vi "Proceed.vi"(7 "component is ready (Y)":bool=TRUE, 8 "error in (no error)":errorcluster, 10 "ProceedMessage":refnum<class "ProceedMessage.lvclass">, 11 "ImageStack in":refnum<class "Invivo_ImageStack.lvclass">) -> (0 "error out":errorcluster, 2 "all observers are ready?":bool, 3 "ImageStack out":refnum<class "Invivo_ImageStack.lvclass">)   [LabVIEW 2012, in "Invivo_ImageStack.lvclass"]
uses:
  Invivo_ImageStack.lvclass
  <vilib>/Distrio/Murmex/ProceedMessage/ProceedMessage.lvclass
  Invivo_ImageStack.lvclass/Invivo_ImageStack.ctl
  <vilib>/Distrio/Murmex/Murmex/Murmex.lvclass
  <vilib>/Distrio/Murmex/Message/Message.lvclass
panel:
  # "This method is called when the PROCEED\ntrigger is sent. \n\nOverride this method when your component needs to\nrespond to this trigger. \n\nCall parent for proper implementation"
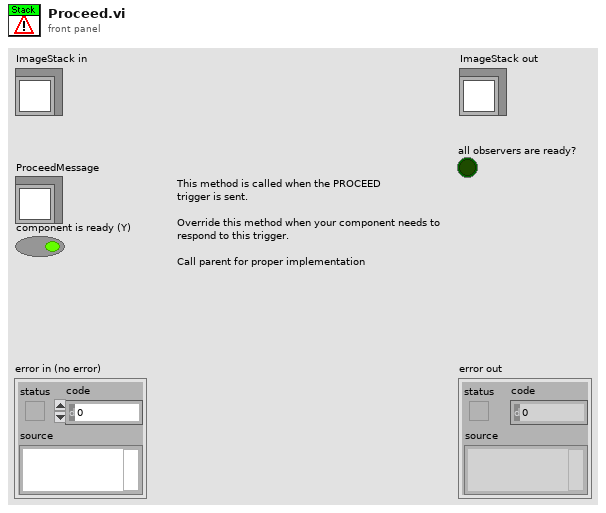
[diagram p1: front panel]
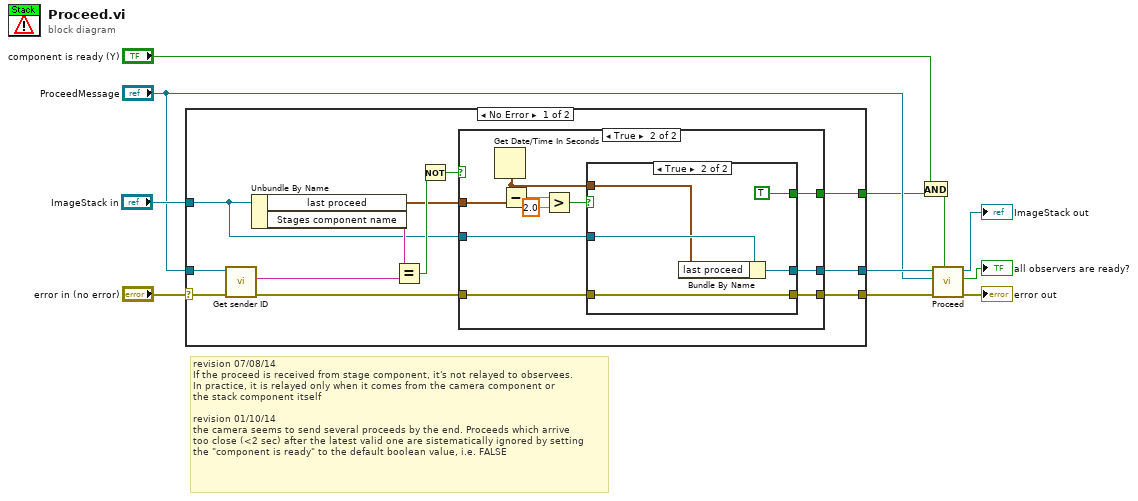
[diagram p0: block diagram]
diagram:
  # "revision 07/08/14\nIf the proceed is received from stage component, it's not relayed to observees.\nIn practice, it is relayed only when it comes from the camera component or \nthe stack component itself\n\nrevision 01/10/14\nthe camera seems to send several proceeds by the end. Proceeds which arrive\ntoo close (<2 sec) after the latest valid one are sistematically ignored by setting\nthe \"component is ready\" to the default boolean value, i.e. FALSE"
  n1 = case shown="No Error" "error in (no error)" {
    selector: "error in (no error)" -> [w22 w43]
    tunnel: "ImageStack in" -> [w15 w44]
    tunnel: [w12 w43] -> w6
    tunnel: [w13 w44] -> w5
    tunnel: "ProceedMessage" -> [w23 _]
    tunnel: [w14 _] -> w3
    frame No Error {
      n2 = call <vilib>:"Get sender ID.vi"("error in (no error)"=w22, "Message in"=w23) -> ("error out"=w17:errorcluster, "sender"=w21:string)  [unwired: 7 in, 1 out]
      n3 = Unbundle By Name(w15) -> ("last proceed"=w16:timestamp, "Stages component name"=w20:string)
      n4 = Equal?(x=w20, y=w21) -> (x = y?=w19:bool)
      n5 = Not(x=w19) -> (.not. x?=w18:bool)
      n6 = case shown="True" w18 {
        tunnel: w17 -> [w24 w26]
        tunnel: w16 -> [_ w35]
        tunnel: w15 -> [w25 w31]
        tunnel: [_ w30] -> w14
        tunnel: [w25 w29] -> w13
        tunnel: [w24 w27] -> w12
        frame False {
        }
        frame True {
          n7 = Get Date/Time In Seconds() -> (seconds since 1Jan1904=w28:timestamp)
          n8 = Subtract(x=w28, y=w35) -> (x-y=w34:dbl)
          n9 = Greater?(x=w34, y=2.0) -> (0:w32:bool)
          n10 = case shown="True" w32 {
            tunnel: w31 -> [w37 w41]
            tunnel: [_ TRUE] -> w30
            tunnel: [w37 w40] -> w29
            tunnel: w28 -> [_ w39]
            tunnel: [w36 w38] -> w27
            tunnel: w26 -> [w36 w38]
            frame False {
            }
            frame True {
              n11 = Bundle By Name(cluster=w41, "last proceed"=w39) -> (w40:refnum<class "Invivo_ImageStack.lvclass">)
            }
          }
        }
      }
    }
    frame Error {
    }
  }
  n12 = And(x="component is ready (Y)", y=w3) -> (x .and. y?=w1:bool)
  n13 = call-parent "Proceed.vi"("component is ready (Y)"=w1, "error in (no error)"=w6, "ProceedMessage"="ProceedMessage", "Murmex in"=w5) -> ("error out"=→"error out":errorcluster, "all observers are ready?"=→"all observers are ready?":bool, "Murmex out"=→"ImageStack out":refnum<class "Invivo_ImageStack.lvclass">)  [unwired: 5 in]
